vi "PixieStopACQ.vi"(8 "error in (no error)":errorcluster) -> (0 "error out":errorcluster)   [LabVIEW 2013]
doc: "Use this template to build a VI to use as a subVI."
uses:
  XIA/Pixie4/Drivers/Pixie4DLL.dll
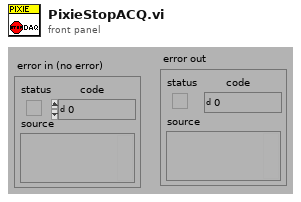
[diagram p1: front panel]
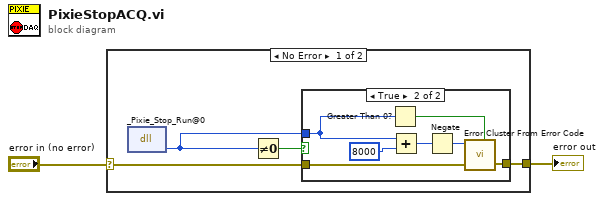
[diagram p0: block diagram]
diagram:
  n1 = case shown="No Error" "error in (no error)" {
    selector: "error in (no error)" -> [w3 w15]
    tunnel: [w4 w15] -> w1
    frame No Error {
      n2 = dll-call lib="C:/XIA/Pixie4/Drivers/Pixie4DLL.dll" fn="_Pixie_Stop_Run@0"() -> ("return type"=w5:i32)  [unwired: 3 in, 2 out]
      n3 = Not Equal To 0?(x=w5) -> (x != 0?=w6:bool)
      n4 = case shown="True" w6 {
        tunnel: w5 -> [_ w14]
        tunnel: [w7 w9] -> w4
        tunnel: w3 -> [w7 w8]
        frame False {
        }
        frame True {
          n5 = Greater Than 0?(x=w14) -> (x > 0?=w11:bool)
          n6 = Add(x=w14, y=8000) -> (x+y=w12:i32)
          n7 = Negate(x=w12) -> (-x=w10:i32)
          n8 = call <vilib>:"Error Cluster From Error Code.vi"("is warning? (False)"=w11, "error in (no error)"=w8, "error code (0)"=w10) -> ("error out"=w9:errorcluster)  [unwired: 1 in, 5 out]
        }
      }
    }
    frame Error {
    }
  }
  "error out" <- w1
